vi "SLT Get Process IDs.vi"(11 "error in (no error)":errorcluster) -> (4 "Process IDs":u32[](array[numeric]), 6 "Number of Processes":u32, 15 "error out":errorcluster)   [LabVIEW 2013, in "ProcessInfo.lvlib"]
doc: "Retrieves the process identifier for each process object in the system."
uses:
  ProcessInfo.lvlib
  psapi.dll
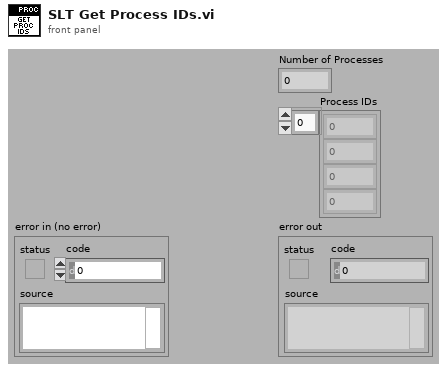
[diagram p1: front panel]
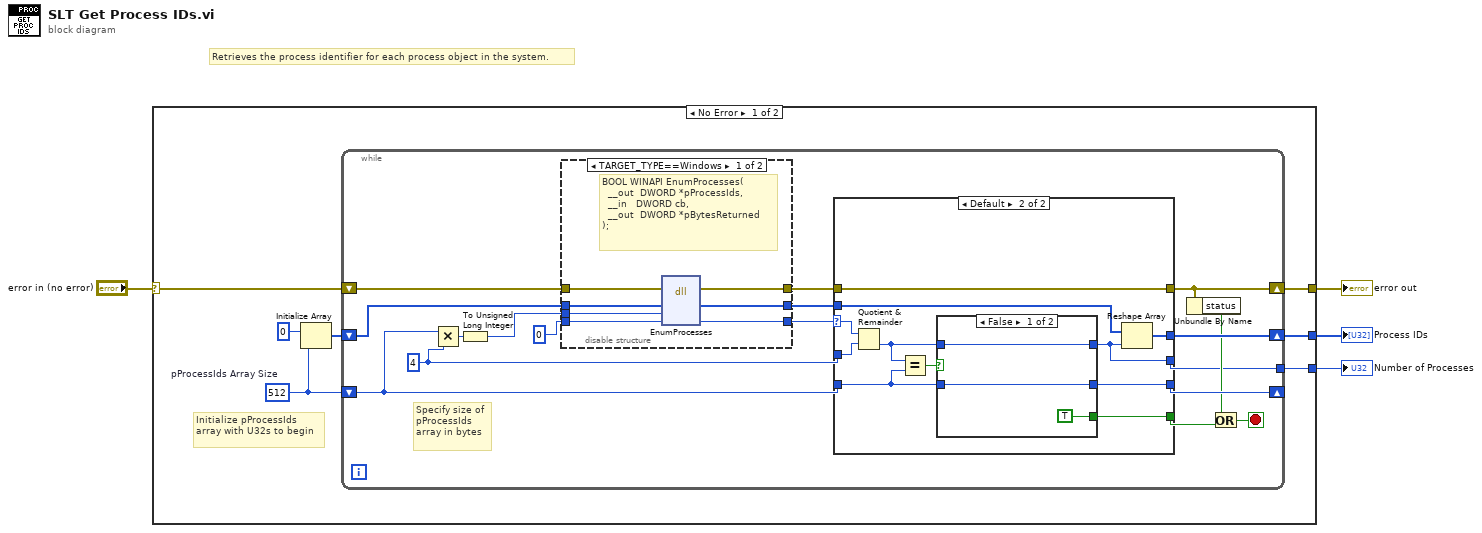
[diagram p0: block diagram]
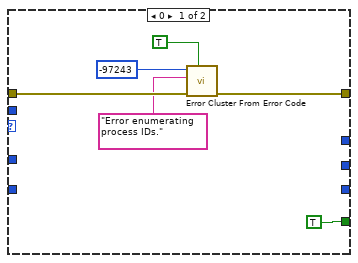
[diagram p3: hidden frame]
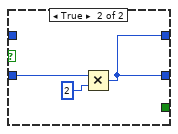
[diagram p4: hidden frame]
diagram:
  # "Retrieves the process identifier for each process object in the system."
  n1 = case shown="No Error" "error in (no error)" {
    selector: "error in (no error)" -> [w5 w62]
    tunnel: [w11 _] -> w4
    tunnel: [w7 w62] -> w3
    tunnel: [w6 _] -> w2
    frame No Error {
      w10 = u32 512  # pProcessIds Array Size
      # "Initialize pProcessIds array with U32s to begin"
      n2 = Initialize Array(u32 0 ("element"), w10) -> (w8:u32[])
      n3 = while {
        shift-right: [w13] -> w7
        shift-left: w5 -> [w25]
        shift-right: [w22] -> _
        shift-left: w10 -> [w23]
        shift-right: [w20] -> w11
        shift-left: w8 -> [w21]
        tunnel: [w12] -> w6
        stop <- w16 stop-if-true
        w24 = u32 4 ("y")
        # "Specify size of pProcessIds array in bytes"
        n4 = Multiply(x=w23, y=w24) -> (x*y=w27:u32)
        n5 = To Unsigned Long Integer(number=w27) -> (unsigned 32bit integer=w26:u32)
        n6 = disable-structure shown="TARGET_TYPE==Windows" {
          disable-tunnel: u32 0 ("y") -> [w35 w36]
          disable-tunnel: w26 -> [w34 _]
          disable-tunnel: w25 -> [w33 w38]
          disable-tunnel: w21 -> [w32 w37]
          disable-tunnel: [w31 w37] -> w19
          disable-tunnel: [w30 w36] -> w17
          disable-tunnel: [w29 w38] -> w14
          frame condition #0 (active) {
            # "BOOL WINAPI EnumProcesses(\n  __out  DWORD *pProcessIds,\n  __in   DWORD cb,\n  __out  DWORD *pBytesReturned\n);"
            n7 = dll-call lib="psapi.dll" fn="EnumProcesses"(error in=w33, "pProcessIds"=w32, "cb"=w34, "pBytesReturned"=w35) -> (error out=w29:errorcluster, "pProcessIds"=w31:u32[], "pBytesReturned"=w30:u32)  [unwired: 3 in, 2 out]
          }
          frame condition #1 {
          }
        }
        n8 = case shown="Default" w17 {
          selector: w17 -> [_ w47]
          tunnel: w24 -> [_ w55]
          tunnel: w23 -> [_ w53]
          tunnel: [_ w52] -> w22
          tunnel: [_ w50] -> w20
          tunnel: w19 -> [_ w49]
          tunnel: [TRUE w48] -> w18
          tunnel: w14 -> [w43 w46]
          tunnel: [w42 w46] -> w13
          tunnel: [_ w45] -> w12
          frame 0 {
            n9 = call <vilib>:"Error Cluster From Error Code.vi"("show call chain? (False)"=TRUE, "error in (no error)"=w43, "error message (\"\")"="Error enumerating process IDs." ("error message (\"\")"), "error code (0)"=-97243) -> ("error out"=w42:errorcluster)  [unwired: 5 in]
          }
          frame Default {
            n10 = Quotient & Remainder(x=w47, y=w55) -> (floor(x/y)=w51:u32)  [unwired: 1 out]
            n11 = Equal?(x=w51, y=w53) -> (x = y?=w54:bool)
            n12 = case shown="False" w54 {
              tunnel: w53 -> [w58 w61]
              tunnel: [w58 w59] -> w52
              tunnel: w51 -> [w57 _]
              tunnel: [w57 w59] -> w45
              tunnel: [TRUE _] -> w48
              frame False {
              }
              frame True {
                n13 = Multiply(x=w61, y=u32 2) -> (x*y=w59:u32)
              }
            }
            n14 = Reshape Array(w49, w45) -> (w50:u32[])
          }
        }
        n15 = Unbundle By Name(w13) -> ("status"=w15:bool)
        n16 = Or(x=w15, y=w18) -> (x .or. y?=w16:bool)
      }
    }
    frame Error {
    }
  }
  "error out" <- w3
  "Process IDs" <- w4
  "Number of Processes" <- w2
